vi "Set.vi"(10 "Value":string, 11 "String in":refnum<class "String.lvclass">) -> (3 "String out":refnum<class "String.lvclass">)   [LabVIEW 2020, in "Conditum.lvlib" / "Columns.lvlib" / "String.lvclass"]
uses:
  String.lvclass
  Type/Type.lvclass
  C:/dev/lv/illuminated-g/lv-conditum/Conditum/Columns/Type/Type.lvclass
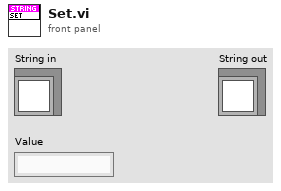
[diagram p1: front panel]
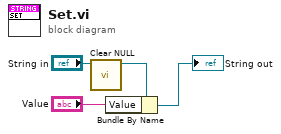
[diagram p0: block diagram]
diagram:
  n1 = call "Clear NULL.vi"("Type in"="String in") -> ("Type out"=w1:refnum<class "String.lvclass">)  [unwired: 10 in]
  n2 = Bundle By Name(cluster=w1, "Value"="Value") -> (→"String out":refnum<class "String.lvclass">)
